vi "Set Background.vi"(8 "error in (no error)":errorcluster, 10 "Background":u32(colorbox), 11 "ArrayManager in":refnum<class "ArrayManager.lvclass">) -> (0 "error out":errorcluster, 3 "ArrayManager out":refnum<class "ArrayManager.lvclass">)   [LabVIEW 2020, in "OOPanel.lvlib" / "ArrayManager.lvclass"]
uses:
  ArrayManager.lvclass
  ArrayManager.lvclass/ArrayManager.ctl
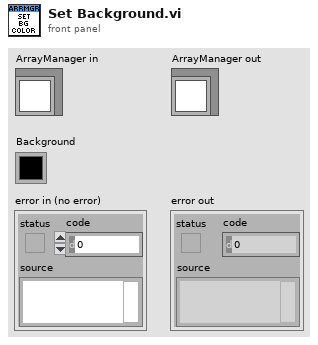
[diagram p1: front panel]
types:
  T1 = typedef "OOPanel.lvlib/ArrayManager.lvclass/State Ref.ctl" = cluster{"Running":bool, "Borders":bool, "Total Height":dbl, "Scroll Visible":bool, "Background":u32}
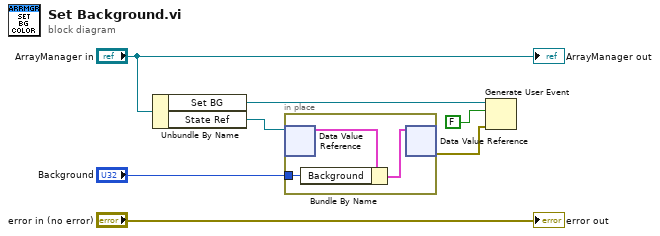
[diagram p0: block diagram]
diagram:
  n1 = Unbundle By Name("ArrayManager in") -> ("Set BG"=w3:refnum<user-event>, "State Ref"=w6:refnum<data-value>)
  n2 = in-place {
    in-place-border: "Background" -> [w8]
    n3 = in-place-dvr #1(w6) -> (w10:T1)  [unwired: 1 out]
    n4 = Bundle By Name(cluster=w10, "Background"=w8) -> (w9:T1)
    n5 = in-place-dvr #1(w9) -> (w2:errorcluster)  [unwired: 1 out]
  }
  n6 = Generate User Event(user event=w3, event data cluster=FALSE ("event data"), error in=w2) -> ()  [unwired: 1 in, 2 out]
  "error out" <- "error in (no error)"
  "ArrayManager out" <- "ArrayManager in"
